vi "TestButton.vi"() -> ()   [LabVIEW 2017]
panel:
  out "Boolean":bool
  in  "OK Button":bool
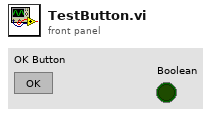
[diagram p1: front panel]
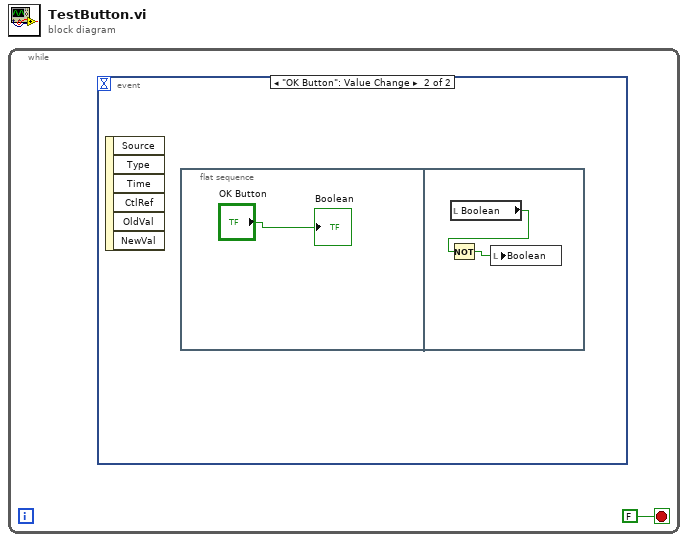
[diagram p0: block diagram]
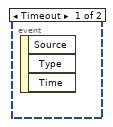
[diagram p2: hidden frame]
diagram:
  n1 = while {
    stop <- FALSE stop-if-true
    n2 = event shown="[1] \"OK Button\": Value Change" {
      selector: _ -> [_ _]
      dyn-events: _ -> [_ _]
      timeout: _ -> [_ _]
      event Timeout {
        n3 = event-data() -> ()  [unwired: 1 in, 3 out]
      }
      event "OK Button": Value Change {
        n4 = event-data() -> ()  [unwired: 1 in, 6 out]
        n5 = flat-sequence {
          frame #0 {
            "Boolean" <- "OK Button"
          }
          frame #1 {
            n6 = local read "Boolean"() -> (w3:bool)
            n7 = Not(x=w3) -> (.not. x?=w4:bool)
            n8 = local write "Boolean"(w4) -> ()
          }
        }
      }
    }
  }
